vi "Update Event Registration.vi"(8 "error in (no error)":errorcluster, 11 "Broadcast Message Receiver in":refnum<class "Broadcast Message Receiver.lvclass">) -> (0 "error out":errorcluster, 3 "Broadcast Message Receiver out":refnum<class "Broadcast Message Receiver.lvclass">)   [LabVIEW 2020, in "Broadcast Message Receiver.lvclass"]
uses:
  Broadcast Message Receiver.lvclass
  <vilib>/Astemes/Triarc Framework/Application/Application.lvclass
  Broadcast Message Receiver.lvclass/Broadcast Message Receiver.ctl
  <vilib>/Astemes/Triarc Framework/Process/Process.lvclass/Process.ctl
  <vilib>/Astemes/Triarc Framework/Process/Public/Lifecycle/Get Lifecycle State.vi
  <vilib>/Utility/error.llb/Clear Errors.vi
  <vilib>/Astemes/Triarc Framework/Application/Protected/Get Broadcast Events Recursively.vi
  <vilib>/Utility/error.llb/Error Cluster From Error Code.vi
  <vilib>/Astemes/Triarc Framework/Process/Process.lvclass
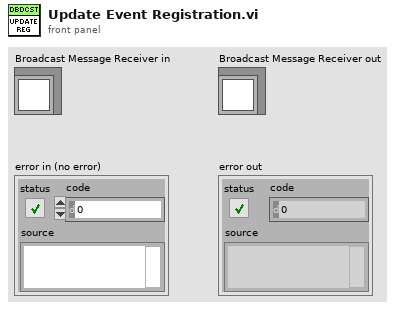
[diagram p1: front panel]
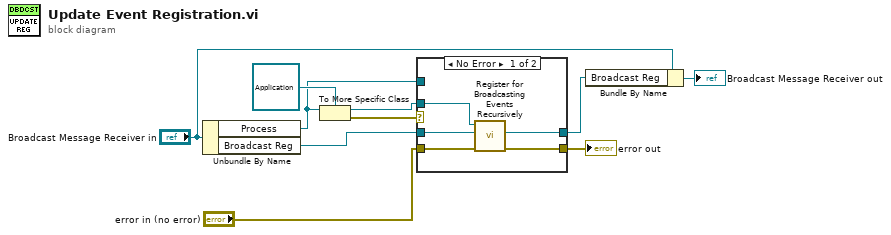
[diagram p0: block diagram]
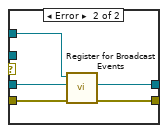
[diagram p2: hidden frame]
diagram:
  n1 = Unbundle By Name("Broadcast Message Receiver in") -> ("Process"=w4:refnum<class "Process.lvclass">, "Broadcast Reg"=w3:refnum<event-registration>)
  n2 = To More Specific Class(target class=refnum<class "Application.lvclass"> refnum ("Application In"), reference=w4) -> (specific class reference=w7:refnum<class "Application.lvclass">, error out=w9:errorcluster)  [unwired: 1 in]
  n3 = case shown="No Error" w9 {
    tunnel: w7 -> [w15 _]
    tunnel: [w14 w19] -> w10
    tunnel: w4 -> [_ w20]
    tunnel: w3 -> [w13 w18]
    tunnel: [w12 w16] -> w2
    tunnel: "error in (no error)" -> [w11 w17]
    frame No Error {
      n4 = call <vilib>:"Register for Broadcasting Events Recursively.vi"("error in (no error)"=w11, "Event Registration Refnum In"=w13, "Application In"=w15) -> ("error out"=w12:errorcluster, "Event Registration Refnum Out"=w14:refnum<event-registration>)  [unwired: 6 in, 1 out]
    }
    frame Error {
      n5 = call <vilib>:"Register for Broadcast Events.vi"("error in (no error)"=w17, "Event Registration Refnum In"=w18, "Process In"=w20) -> ("error out"=w16:errorcluster, "Event Registration Refnum Out"=w19:refnum<event-registration>)  [unwired: 6 in, 1 out]
    }
  }
  "error out" <- w2
  n6 = Bundle By Name(cluster="Broadcast Message Receiver in", "Broadcast Reg"=w10) -> (→"Broadcast Message Receiver out":refnum<class "Broadcast Message Receiver.lvclass">)
